vi "PassThru.vi"(8 "error in (no error)":errorcluster, 9 "timeout ms (1000)":i32=1000, 10 "Cmd":cluster{"cmd":u8[], "require response?":bool}={"cmd"=[], "require response?"=TRUE}, 11 "Ref":T1) -> (0 "error out":errorcluster, 2 "Resp":T5, 3 "Ref out":T1)   [LabVIEW 2019, in "Diagnostics Host Automation API.lvlib"]
uses:
  Diagnostics Host Automation API.lvlib
  Addon/Addon Shared/Types/HostAutomation.Ref.ctl
  <vilib>/NI/STM/TCP/TCP Connection Info.ctl
  <vilib>/NI/STM/SubVIs/MetaDataElement.ctl
  Addon/Addon Shared/Types/DTC.Codes.ctl
  <vilib>/NI/NI VeriStand Addon Network Comm/Shared/NI VeriStand Addon Network Comm Shared.lvlib
  <vilib>/NI/STM/NI STM.lvlib
  Addon/Addon Shared/Diagnostics Addon Shared.lvlib
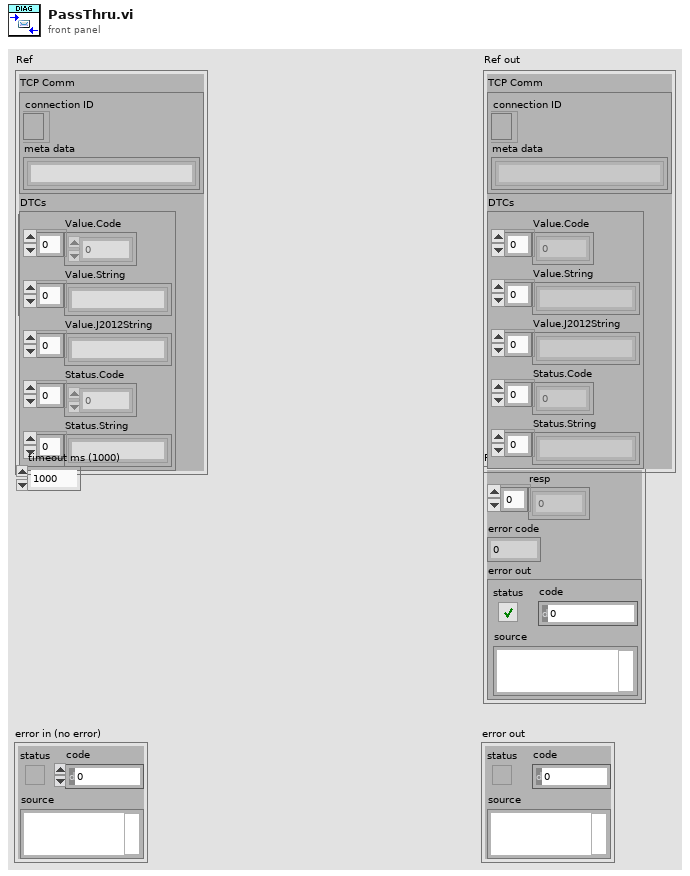
[diagram p1: front panel]
types:
  T1 = typedef "Diagnostics Addon Shared.lvlib/HostAutomation.Ref.ctl" = cluster{"TCP Comm":T2, "DTCs":T4}
  T2 = typedef "NI STM.lvlib/TCP Connection Info.ctl" = cluster{"connection ID":refnum<k5>, "meta data":T3[]}
  T3 = typedef "NI STM.lvlib/MetaDataElement.ctl" = string
  T4 = typedef "Diagnostics Addon Shared.lvlib/DTC.Codes.ctl" = cluster{"Value.Code":dbl[], "Value.String":string[], "Value.J2012String":string[], "Status.Code":dbl[], "Status.String":string[]}
  T5 = cluster{"resp":u8[], "error code":u8, "error out":errorcluster}
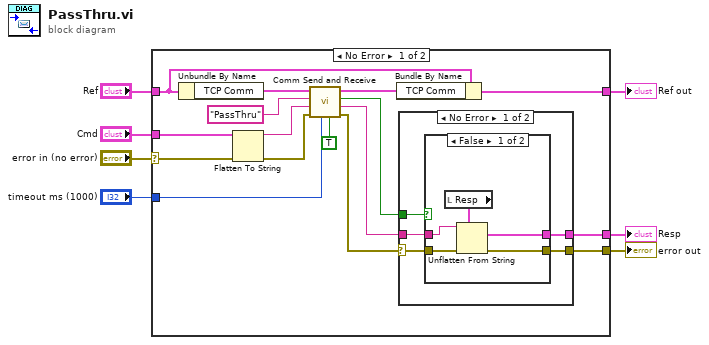
[diagram p0: block diagram]
diagram:
  n1 = case shown="No Error" "error in (no error)" {
    selector: "error in (no error)" -> [w22 w37]
    tunnel: "Ref" -> [w10 w36]
    tunnel: [w8 w36] -> w6
    tunnel: [w23 w37] -> w5
    tunnel: "timeout ms (1000)" -> [w12 _]
    tunnel: "Cmd" -> [w21 _]
    tunnel: [w20 _] -> w1
    frame No Error {
      n2 = Unbundle By Name(w10) -> ("TCP Comm"=w11:T2)
      n3 = Flatten To String(anything=w21, error in (no error)=w22) -> (data string=w14:string, error out=w15:errorcluster)  [unwired: 2 in, 1 out]
      n4 = call <vilib>:"Comm Send and Receive.vi"("Resp Required?"=TRUE, "Timeout (ms)"=w12, "error in (no error)"=w15, "Data"=w14, "Name"="PassThru", "connection info"=w11) -> ("error out"=w16:errorcluster, "Data"=w17:string, "Timed Out?"=w18:bool, "connection info"=w9:T2)  [unwired: 2 in]
      n5 = Bundle By Name(cluster=w10, "TCP Comm"=w9) -> (w8:T1)
      n6 = case shown="No Error" w16 {
        selector: w16 -> [w26 w35]
        tunnel: w18 -> [w28 _]
        tunnel: [w27 w35] -> w23
        tunnel: w17 -> [w25 _]
        tunnel: [w24 _] -> w20
        frame No Error {
          n7 = case shown="False" w28 {
            tunnel: [w30 w34] -> w27
            tunnel: w26 -> [w31 w34]
            tunnel: w25 -> [w32 _]
            tunnel: [w29 _] -> w24
            frame False {
              n8 = local read "Resp"() -> (w33:T5)
              n9 = Unflatten From String(type=w33, binary string=w32, error in (no error)=w31) -> (value=w29:T5, error out=w30:errorcluster)  [unwired: 2 in, 1 out]
            }
            frame True {
            }
          }
        }
        frame Error {
        }
      }
    }
    frame Error {
    }
  }
  "Ref out" <- w6
  "error out" <- w5
  "Resp" <- w1
